vi "Open_File.vi"(5 "Message?":bool, 7 "Path in":path, 8 "error in (no error)":errorcluster, 9 "Sequence in":string[](array[string]), 10 "Buffer in":string[](array[string]), 11 "Sequence Caption in":string) -> (0 "error out":errorcluster, 1 "Sequence out":string[](array[string]), 2 "Buffer out":string[](array[string]), 3 "Sequence Caption out":string, 4 "Path out":path, 6 "top row":i32)   [LabVIEW 2019]
uses:
  <vilib>/Utility/file.llb/Write To Spreadsheet File (string).vi
  <vilib>/Utility/file.llb/Read From Spreadsheet File (string).vi
panel:
  # "to determine vertical scroll bar"
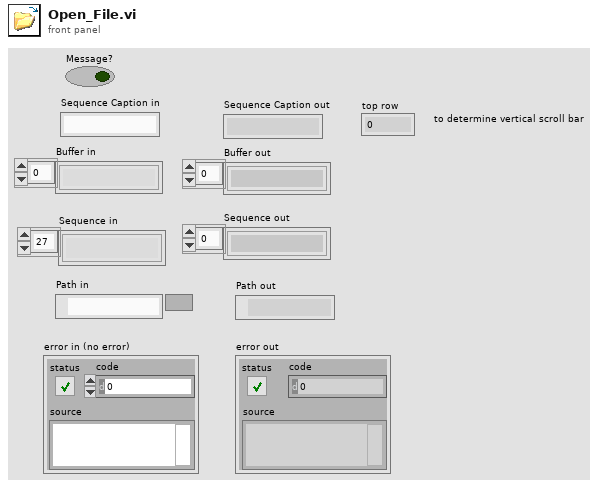
[diagram p1: front panel]
types:
  T1 = enum16{"Left Button", "Center Button", "Right Button", "Window Close"}
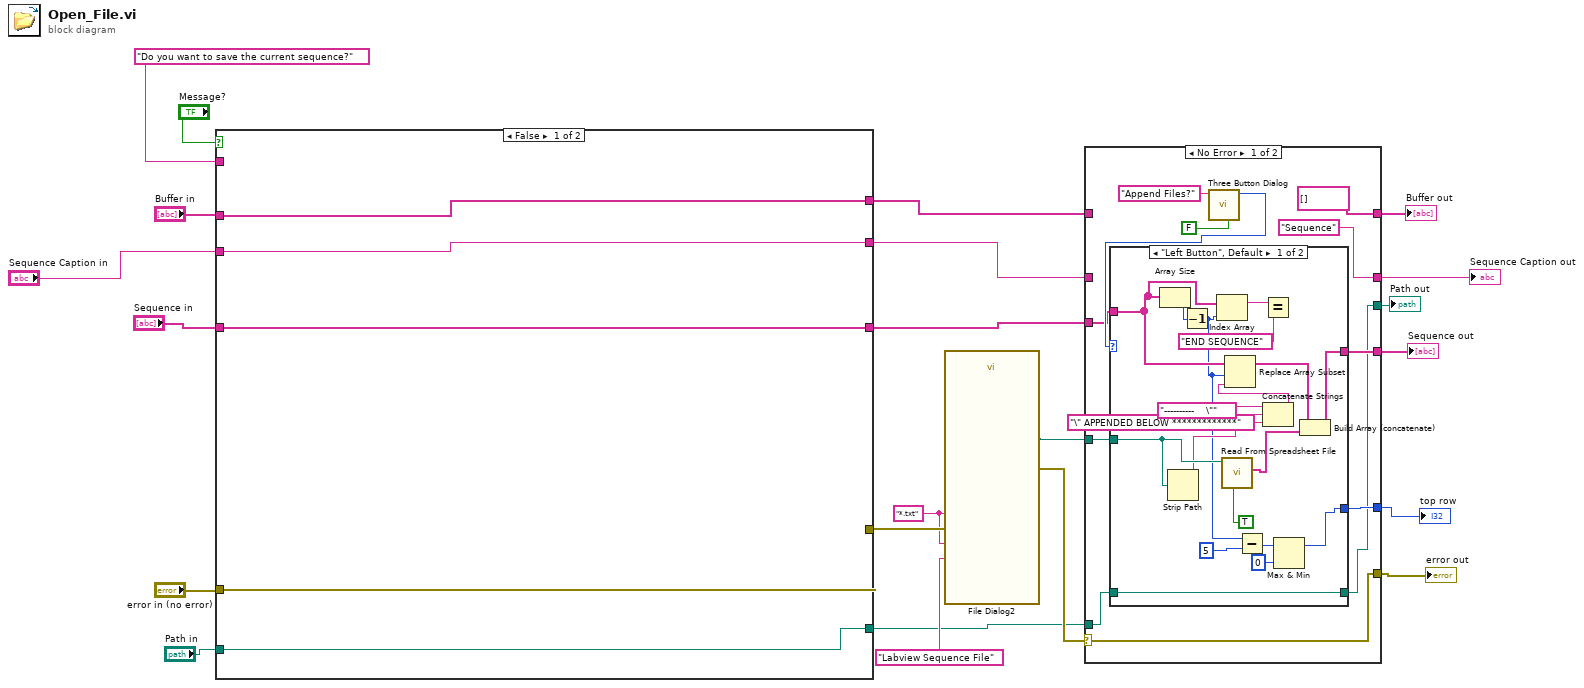
[diagram p0: block diagram]
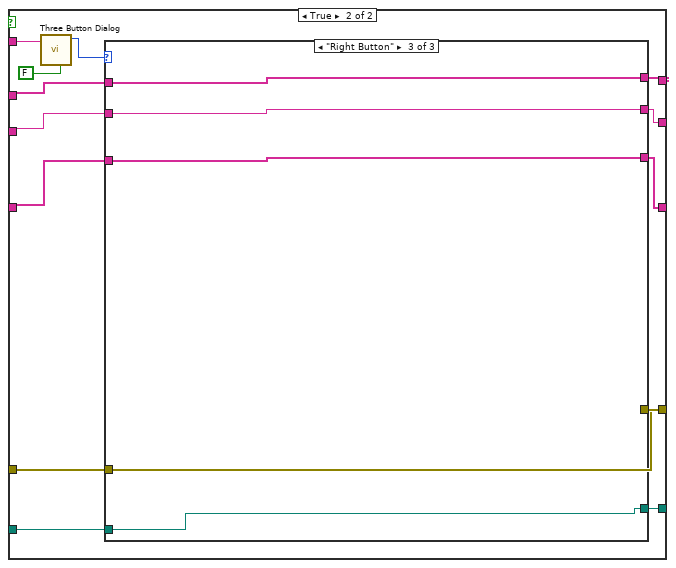
[diagram p2: hidden frame]
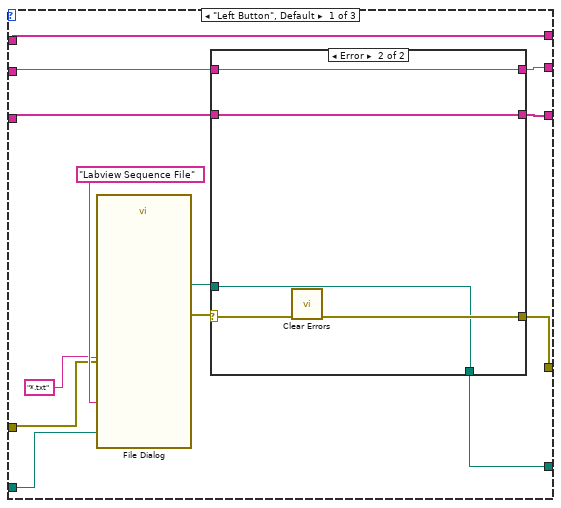
[diagram p3: hidden frame]
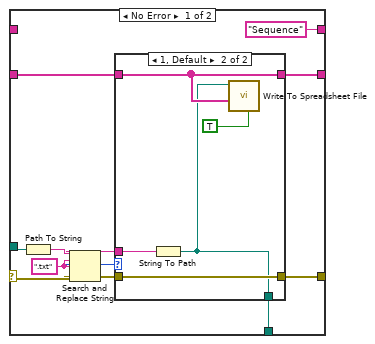
[diagram p4: hidden frame]
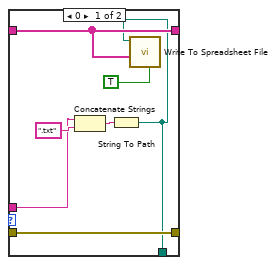
[diagram p5: hidden frame]
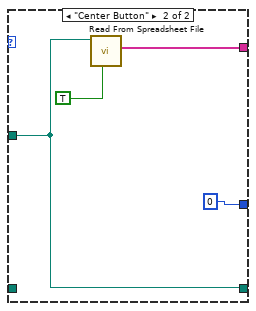
[diagram p7: hidden frame]
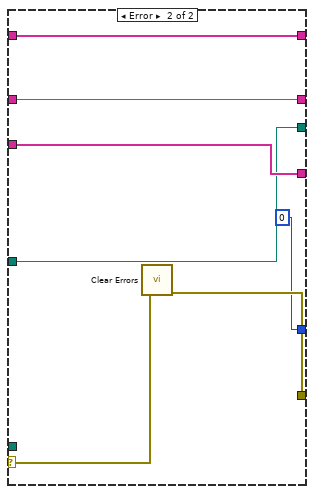
[diagram p8: hidden frame]
diagram:
  w17 = "*.txt"
  n1 = case shown="False" "Message?" {
    tunnel: "error in (no error)" -> [w24 w40]
    tunnel: "Sequence in" -> [w25 w39]
    tunnel: "Path in" -> [w23 w38]
    tunnel: [w24 w37] -> w19
    tunnel: "Buffer in" -> [w27 w36]
    tunnel: [w25 w35] -> w12
    tunnel: [w27 w34] -> w11
    tunnel: "Sequence Caption in" -> [w26 w33]
    tunnel: [w26 w32] -> w7
    tunnel: "Do you want to save the current sequence?" ("message") -> [_ w29]
    tunnel: [w23 w28] -> w1
    frame False {
    }
    frame True {
      n2 = call <vilib>:"Three Button Dialog.vi"("Allow user to close window? (TRUE)"=FALSE, "message"=w29) -> ("Which Button?"=w31:T1)  [unwired: 9 in]
      n3 = case shown="\"Right Button\"" w31 {
        tunnel: w40 -> [w51 w87 w92]
        tunnel: w39 -> [w49 w86 w90]
        tunnel: w38 -> [w48 w83 w88]
        tunnel: [w46 w87 w92] -> w37
        tunnel: w36 -> [w45 w85 w91]
        tunnel: [w45 w85 w91] -> w34
        tunnel: [w44 w86 w90] -> w35
        tunnel: [w43 w84 w89] -> w32
        tunnel: w33 -> [w42 w84 w89]
        tunnel: [w41 w83 w88] -> w28
        frame "Left Button", Default {
          n4 = call "File Dialog"("start path"=w48, "default name"="*.txt", "error in"=w51, "pattern label"="Labview Sequence File") -> ("selected path"=w47:path, "error out"=w50:errorcluster)  [unwired: 8 in, 2 out]
          n5 = case shown="Error" w50 {
            selector: w50 -> [w62 w80]
            tunnel: w49 -> [w65 w82]
            tunnel: w47 -> [w61 w78]
            tunnel: [w57 w79] -> w46
            tunnel: [w56 w82] -> w44
            tunnel: ["Sequence" ("pattern label") w81] -> w43
            tunnel: w42 -> [_ w81]
            tunnel: [w54 w78] -> w41
            frame No Error {
              w63 = ".txt" ("search string")
              n6 = Path To String(path=w61) -> (string=w64:string)
              n7 = Search and Replace String(input string=w64, search string=w63, replace string=w63, error in=w62) -> (result string=w59:string, number of replacements=w60:i32, error out=w58:errorcluster)  [unwired: 4 in, 1 out]
              n8 = case shown="1, Default" w60 {
                tunnel: w65 -> [w67 w74]
                tunnel: w59 -> [w70 w76]
                tunnel: w58 -> [w68 w75]
                tunnel: [w68 w75] -> w57
                tunnel: [w67 w74] -> w56
                tunnel: [w66 w73] -> w54
                frame 0 {
                  n9 = Concatenate Strings(w70, ".txt" ("string")) -> (w71:string)
                  n10 = String To Path(string=w71) -> (path=w66:path)
                  n11 = call-poly <vilib>:"Write To Spreadsheet File.vi"("transpose? (no:F)"=TRUE, "1D data"=w67, "file path (dialog if empty)"=w66) -> ()  [unwired: 5 in, 1 out]
                }
                frame 1, Default {
                  n12 = String To Path(string=w76) -> (path=w73:path)
                  n13 = call-poly <vilib>:"Write To Spreadsheet File.vi"("transpose? (no:F)"=TRUE, "1D data"=w74, "file path (dialog if empty)"=w73) -> ()  [unwired: 5 in, 1 out]
                }
              }
            }
            frame Error {
              n14 = call <vilib>:"Clear Errors.vi"("error in (no error)"=w80) -> ("error out"=w79:errorcluster)  [unwired: 5 in, 1 out]
            }
          }
        }
        frame "Center Button" {
        }
        frame "Right Button" {
        }
      }
    }
  }
  n15 = call "File Dialog2"("default name"=w17, "error in"=w19, "pattern (all files)"=w17, "pattern label"="Labview Sequence File") -> ("selected path"=w15:path, "error out"=w14:errorcluster)  [unwired: 8 in, 2 out]
  n16 = case shown="No Error" w14 {
    selector: w14 -> [w103 w130]
    tunnel: w15 -> [w101 w131]
    tunnel: [w104 w134] -> w13
    tunnel: w12 -> [w96 w134]
    tunnel: w11 -> [_ w133]
    tunnel: [string[] [] ("Buffer in") w133] -> w10
    tunnel: [w103 w129] -> w9
    tunnel: w7 -> [_ w132]
    tunnel: ["Sequence" ("pattern label") w132] -> w6
    tunnel: [w94 w131] -> w5
    tunnel: [w95 0] -> w2
    tunnel: w1 -> [w93 _]
    frame No Error {
      n17 = call <vilib>:"Three Button Dialog.vi"("Allow user to close window? (TRUE)"=FALSE, "message"="Append Files?") -> ("Which Button?"=w98:T1)  [unwired: 9 in]
      n18 = case shown="\"Left Button\", Default" w98 {
        tunnel: [w121 w126] -> w104
        tunnel: w101 -> [w114 w124]
        tunnel: w96 -> [w120 _]
        tunnel: [w106 0] -> w95
        tunnel: [w105 w124] -> w94
        tunnel: w93 -> [w105 _]
        frame "Left Button", Default {
          n19 = Array Size(array=w120) -> (size(s)=w119:i32)
          n20 = Strip Path(path=w114) -> (name=w113:string)  [unwired: 1 out]
          n21 = Decrement(x=w119) -> (x-1=w108:i32)
          n22 = Index Array(array=w120, index=w108) -> (element=w118:string)
          n23 = call-poly <vilib>:"Read From Spreadsheet File.vi"("transpose (no:F)"=TRUE, "file path (dialog if empty)"=w114) -> ("first row"=w122:string[])  [unwired: 5 in, 4 out]
          n24 = Subtract(x=w108, y=5) -> (x-y=w109:i32)
          n25 = Equal?(x=w118, y="END SEQUENCE") -> ()  [unwired: 1 out]
          n26 = Concatenate Strings("----------    \"" ("y"), w113, "\" APPENDED BELOW *************" ("string")) -> (w112:string)
          n27 = Replace Array Subset(array=w120, new element=w112, index=w108) -> (w116:string[])
          n28 = Max & Min(x=w109, y=0) -> (max(x,y)=w106:i32)  [unwired: 1 out]
          n29 = Build Array (concatenate)(w116, w122) -> (w121:string[])
        }
        frame "Center Button" {
          n30 = call-poly <vilib>:"Read From Spreadsheet File.vi"("transpose (no:F)"=TRUE, "file path (dialog if empty)"=w124) -> ("first row"=w126:string[])  [unwired: 5 in, 4 out]
        }
      }
    }
    frame Error {
      n31 = call <vilib>:"Clear Errors.vi"("error in (no error)"=w130) -> ("error out"=w129:errorcluster)  [unwired: 5 in, 1 out]
    }
  }
  "Buffer out" <- w10
  "Sequence out" <- w13
  "Sequence Caption out" <- w6
  "Path out" <- w5
  "error out" <- w9
  "top row" <- w2
